vi "Read Bacta [l].vi"(8 "error in (no error)":errorcluster, 11 "MedicalDroid in":refnum<class "MedicalDroid.lvclass">) -> (0 "error out":errorcluster, 2 "Bacta [l]":u8 max=10, 3 "MedicalDroid out":refnum<class "MedicalDroid.lvclass">)   [LabVIEW 2021, in "MedicalDroid.lvclass"]
uses:
  MedicalDroid.lvclass
  MedicalDroid.lvclass/MedicalDroid.ctl
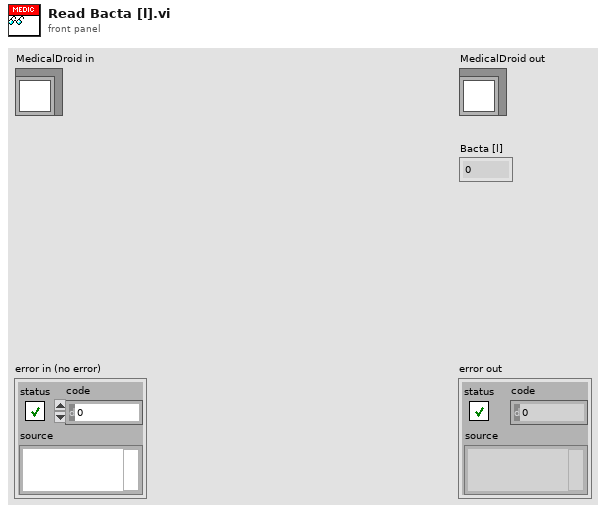
[diagram p1: front panel]
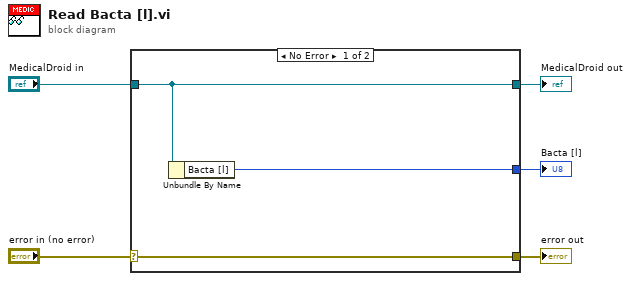
[diagram p0: block diagram]
diagram:
  n1 = case shown="No Error" "error in (no error)" {
    selector: "error in (no error)" -> [w8 w9]
    tunnel: [w8 w9] -> w4
    tunnel: [w7 w10] -> w2
    tunnel: "MedicalDroid in" -> [w7 w10]
    tunnel: [w6 _] -> w1
    frame No Error {
      n2 = Unbundle By Name(w7) -> ("Bacta [l]"=w6:u8)
    }
    frame Error {
    }
  }
  "error out" <- w4
  "MedicalDroid out" <- w2
  "Bacta [l]" <- w1
